vi "New.vi"(11 "VISA resource name":refnum<visa-resource-name>) -> (0 "error out":errorcluster, 3 "AlphaStep One out":refnum<class "AlphaStep One.lvclass">)   [LabVIEW 2018, in "AlphaStep One.lvclass"]
uses:
  AlphaStep One.lvclass
  AlphaStep One.lvclass/AlphaStep One.ctl
  Serial Device/Serial Device.lvclass
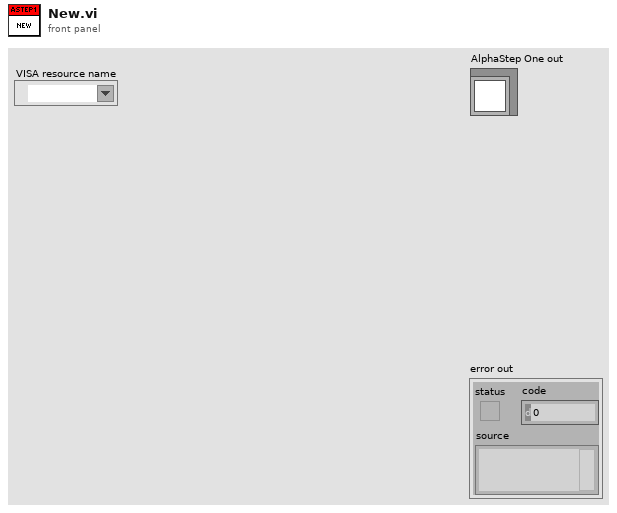
[diagram p1: front panel]
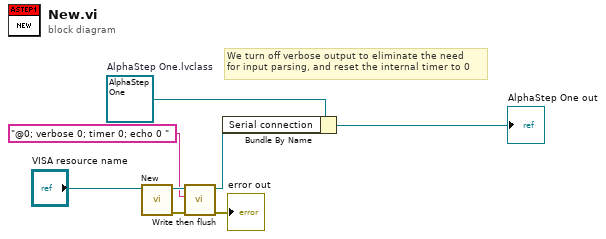
[diagram p0: block diagram]
diagram:
  w8 = refnum<class "AlphaStep One.lvclass"> refnum  # AlphaStep One.lvclass
  # "We turn off verbose output to eliminate the need\nfor input parsing, and reset the internal timer to 0"
  n1 = call "New.vi"("VISA resource name"="VISA resource name") -> ("error out"=w4:errorcluster, "Serial Device out"=w6:refnum<class "Serial Device.lvclass">)  [unwired: 9 in]
  n2 = call "Write then flush.vi"("error in (no error)"=w4, "TX Data"="@0; verbose 0; timer 0; echo 0 ", "Serial Device in"=w6) -> ("error out"=→"error out":errorcluster, "Serial Device out"=w2:refnum<class "Serial Device.lvclass">)  [unwired: 7 in]
  n3 = Bundle By Name(cluster=w8, "Serial connection"=w2) -> (→"AlphaStep One out":refnum<class "AlphaStep One.lvclass">)
